vi "StateMacines_old.vi"(5 "PWM Demand":i32, 6 "Operate":bool, 7 "Purge Time":i32=10, 8 "PWMStart":i32, 9 "broadcasts":variant, 10 "CurrentPWM":i32, 11 "Inputs":T1) -> (0 "StopOperation":bool, 1 "Opis":string, 2 "DKG":bool, 3 "DisableStartBtn":bool)   [LabVIEW 2015]
uses:
  Typedefs/mqttinputs.ctl
  Typedefs/DKGSMin.ctl
  Libraries/MQTT.lvlibp
panel:
  in  "error out 2":errorcluster
  out "error out":errorcluster
  in  "Module ID":i32=-1
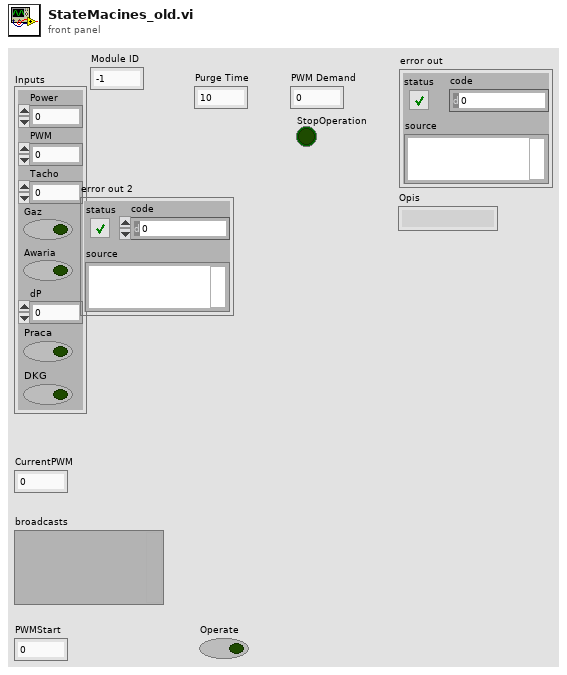
[diagram p1: front panel]
types:
  T1 = typedef "mqttinputs.ctl" = cluster{"Power":dbl, "PWM":i32, "Tacho":i32, "Gaz":bool, "Awaria":bool, "dP":dbl, "Praca":bool, "DKG":bool}
  T2 = cluster{"PWM":i32, "PurgeStart":bool, "DKG":bool, "Purge Time":i32}
  T3 = typedef "DKGSMin.ctl" = cluster{"Lockout":bool, "Operate":bool, "V1":bool, "PurgeTime":dbl, "Burning":bool, "PWM":i32, "PWMStart":i32, "SettleTime(s)":dbl, "DKG":bool}
  T4 = typedef "DKGSMOut.ctl" = cluster{"DisableStartBtn":bool, "Kasawar":bool, "DKG":bool, "PWM":i32, "Purge":bool, "Opis":string, "StopOperation":bool}
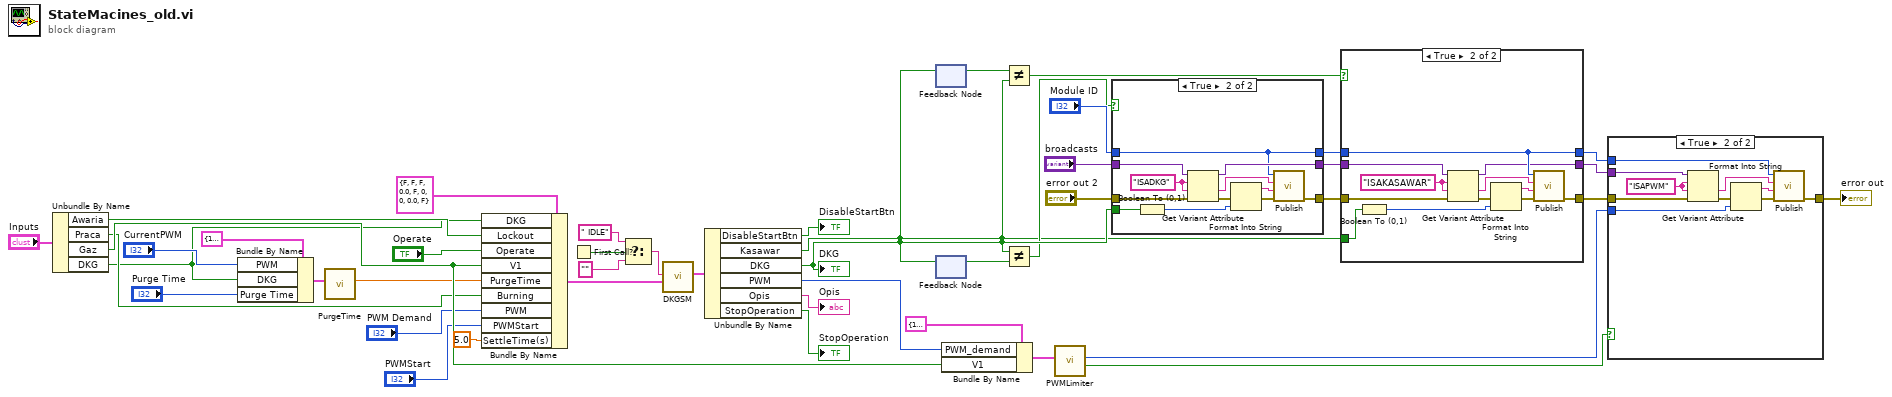
[diagram p0: block diagram]
diagram:
  n1 = Unbundle By Name("Inputs") -> ("Awaria"=w43:bool, "Praca"=w16:bool, "Gaz"=w44:bool, "DKG"=w2:bool)
  n2 = Bundle By Name(cluster=T2 {"PWM"=100, "PurgeStart"=FALSE, "DKG"=FALSE, "Purge Time"=60} ("Cluster"), "PWM"="CurrentPWM", "DKG"=w2, "Purge Time"="Purge Time") -> (w39:T2)
  n3 = call "PurgeTime.vi"("Cluster"=w39) -> ("Purge Time"=w36:dbl)  [unwired: 10 in]
  n4 = Bundle By Name(cluster=T3 {"Lockout"=FALSE, "Operate"=FALSE, "V1"=FALSE, "PurgeTime"=0.0, "Burning"=FALSE, "PWM"=0, "PWMStart"=0, "SettleTime(s)"=0.0, "DKG"=FALSE} ("input"), "DKG"=w2, "Lockout"=w43, "Operate"="Operate", "V1"=w44, "PurgeTime"=w36, "Burning"=w16, "PWM"="PWM Demand", "PWMStart"="PWMStart", "SettleTime(s)"=5.0) -> (w33:T3)
  n5 = First Call?() -> (First Call?: T/F=w7:bool)
  n6 = Select(t=" IDLE", s=w7, f="") -> (s? t:f=w4:string)
  n7 = call "DKGSM.vi"("input"=w33, "State"=w4) -> ("DKGSMOutput"=w34:T4)  [unwired: 9 in]
  n8 = Unbundle By Name(w34) -> ("DisableStartBtn"=→"DisableStartBtn":bool, "Kasawar"=w22:bool, "DKG"=w27:bool, "PWM"=w35:i32, "Opis"=→"Opis":string, "StopOperation"=→"StopOperation":bool)
  "DKG" <- w27
  n9 = feedback #1() -> (w40:bool)  [unwired: 1 in]
  n10 = feedback-in #1(w22) -> ()
  n11 = feedback #2() -> (w41:bool)  [unwired: 1 in]
  n12 = feedback-in #2(w27) -> ()
  n13 = Bundle By Name(cluster=cluster{"PWM_demand":i32, "V1":bool} {"PWM_demand"=100, "V1"=TRUE} ("Cluster"), "PWM_demand"=w35, "V1"=w44) -> (w31:cluster{"PWM_demand":i32, "V1":bool})
  n14 = Not Equal?(x=w40, y=w22) -> (x != y?=w23:bool)
  n15 = Not Equal?(x=w27, y=w41) -> (x != y?=w26:bool)
  n16 = call "PWMLimiter.vi"("Cluster"=w31) -> ("Boolean"=w10:bool, "PWM"=w9:i32)  [unwired: 9 in]
  n17 = case shown="True" w26 {
    tunnel: "broadcasts" -> [w48 w60]
    tunnel: "Module ID" -> [w47 w52]
    tunnel: w27 -> [_ w57]
    tunnel: [w48 w53] -> w25
    tunnel: [w47 w52] -> w24
    tunnel: [w46 w50] -> w21
    tunnel: "error out 2" -> [w46 w49]
    frame False {
    }
    frame True {
      w58 = "ISADKG" ("name")
      n18 = Boolean To (0,1)(Boolean=w57) -> (0, 1=w55:i16)
      n19 = Get Variant Attribute(Variant=w60, name=w58, default value (empty Variant)=w58, error in=w49) -> (duplicate Variant=w53:variant, value=w59:string, error out=w51:errorcluster)  [unwired: 1 out]
      n20 = Format Into String(error in=w51, w55) -> (resulting string=w54:string, error out=w56:errorcluster)  [unwired: 2 in]
      n21 = call "Publish.vi"("error in (no error)"=w56, "Payload"=w54, "Topic"=w59, "Module ID"=w52) -> ("error out"=w50:errorcluster)  [unwired: 7 in]
    }
  }
  n22 = case shown="True" w23 {
    tunnel: w24 -> [w62 w65]
    tunnel: w22 -> [_ w73]
    tunnel: w25 -> [w61 w69]
    tunnel: w21 -> [w63 w68]
    tunnel: [w63 w66] -> w13
    tunnel: [w62 w65] -> w12
    tunnel: [w61 w64] -> w11
    frame False {
    }
    frame True {
      w74 = "ISAKASAWAR" ("name")
      n23 = Boolean To (0,1)(Boolean=w73) -> (0, 1=w71:i16)
      n24 = Get Variant Attribute(Variant=w69, name=w74, default value (empty Variant)=w74, error in=w68) -> (duplicate Variant=w64:variant, value=w75:string, error out=w67:errorcluster)  [unwired: 1 out]
      n25 = Format Into String(error in=w67, w71) -> (resulting string=w70:string, error out=w72:errorcluster)  [unwired: 2 in]
      n26 = call "Publish.vi"("error in (no error)"=w72, "Payload"=w70, "Topic"=w75, "Module ID"=w65) -> ("error out"=w66:errorcluster)  [unwired: 7 in]
    }
  }
  n27 = case shown="True" w10 {
    tunnel: w12 -> [_ w86]
    tunnel: w11 -> [_ w81]
    tunnel: w13 -> [w76 w80]
    tunnel: [w76 w78] -> w8
    tunnel: w9 -> [_ w77]
    frame False {
    }
    frame True {
      w84 = "ISAPWM" ("name")
      n28 = Get Variant Attribute(Variant=w81, name=w84, default value (empty Variant)=w84, error in=w80) -> (value=w85:string, error out=w79:errorcluster)  [unwired: 2 out]
      n29 = Format Into String(error in=w79, w77) -> (resulting string=w82:string, error out=w83:errorcluster)  [unwired: 2 in]
      n30 = call "Publish.vi"("error in (no error)"=w83, "Payload"=w82, "Topic"=w85, "Module ID"=w86) -> ("error out"=w78:errorcluster)  [unwired: 7 in]
    }
  }
  "error out" <- w8
